vi "Parse Global Options.vi"(10 "Args in":string[](array[string])) -> (2 "Remaining Args":string[](array[string]), 3 "Global Options":T1)   [LabVIEW 2020, in "GPackTools.lvlib" / "GPackCLI.lvclass"]
uses:
  GPackCLI.lvclass
  Global Options.ctl
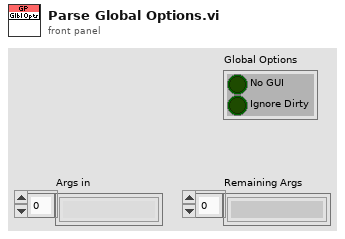
[diagram p1: front panel]
types:
  T1 = typedef "GPackTools.lvlib/GPackCLI.lvclass/Global Options.ctl" = cluster{"No GUI":bool, "Ignore Dirty":bool}
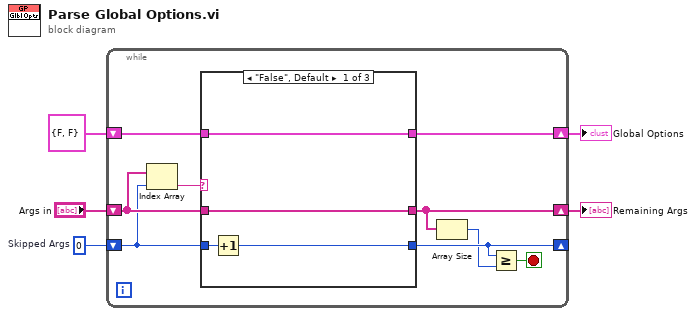
[diagram p0: block diagram]
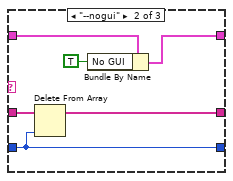
[diagram p2: hidden frame]
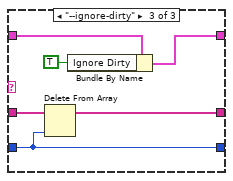
[diagram p3: hidden frame]
diagram:
  w2 = 0  # Skipped Args
  n1 = while {
    shift-right: [w11] -> w4
    shift-left: T1 {"No GUI"=FALSE, "Ignore Dirty"=FALSE} ("Global Options") -> [w14]
    shift-right: [w8] -> _
    shift-left: w2 -> [w10]
    shift-right: [w9] -> w1
    shift-left: "Args in" -> [w12]
    stop <- w6 stop-if-true
    n2 = Index Array(array=w12, index=w10) -> (element=w13:string)
    n3 = case shown="\"False\", Default" w13 {
      tunnel: w14 -> [w16 w24 w30]
      tunnel: w12 -> [w17 w21 w27]
      tunnel: [w16 w22 w29] -> w11
      tunnel: w10 -> [w18 w19 w25]
      tunnel: [w17 w20 w26] -> w9
      tunnel: [w15 w19 w25] -> w8
      frame "False", Default {
        n4 = Increment(x=w18) -> (x+1=w15:i32)
      }
      frame "--nogui" {
        n5 = Delete From Array(array=w21, index=w19) -> (array with subset deleted=w20:string[])  [unwired: 1 in, 1 out]
        n6 = Bundle By Name(cluster=w24, "No GUI"=TRUE) -> (w22:T1)
      }
      frame "--ignore-dirty" {
        n7 = Delete From Array(array=w27, index=w25) -> (array with subset deleted=w26:string[])  [unwired: 1 in, 1 out]
        n8 = Bundle By Name(cluster=w30, "Ignore Dirty"=TRUE) -> (w29:T1)
      }
    }
    n9 = Array Size(array=w9) -> (size(s)=w7:i32)
    n10 = Greater Or Equal?(x=w8, y=w7) -> (x >= y?=w6:bool)
  }
  "Global Options" <- w4
  "Remaining Args" <- w1
